vi "KillCamera.vi"(11 "Camera":T1) -> ()   [LabVIEW 2015]
uses:
  ROS/Code/SubVIs/BaxterCamera.ctl
  ROS/Code/_ROSDefinition.vi
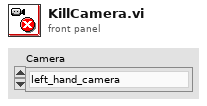
[diagram p1: front panel]
types:
  T1 = typedef "BaxterCamera.ctl" = enum16{"left_hand_camera", "right_hand_camera", "head_camera"}
  T2 = typedef "_ROSControl.ctl" = cluster{"topic port":u16, "Node":string, "topic":string, "type":string, "node port":u16, "error ":errorcluster, "Direction":T3, "Update (ms)":u16, "FIFO size":u16}
  T3 = typedef "_ROSDirection.ctl" = enum16{"Node", "Publisher", "Subscriber", "ServiceClient", "ServiceProvider"}
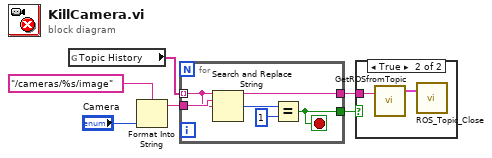
[diagram p0: block diagram]
diagram:
  n1 = global read "_ROSDefinition.vi" "Topic History"() -> (w3:string[])
  n2 = Format Into String(format string="/cameras/%s/image" ("topic"), "Camera") -> (resulting string=w4:string)  [unwired: 2 in, 1 out]
  n3 = for {
    tunnel: w3 -> [w11] mode=indexing
    tunnel: w4 -> [w12]
    tunnel: [w8] -> w5
    tunnel: [w7] -> w6
    stop <- w7 stop-if-true
    n4 = Search and Replace String(input string=w11, search string=w12, replace string=w11) -> (result string=w8:string, number of replacements=w10:i32)  [unwired: 5 in, 2 out]
    n5 = Equal?(x=w10, y=1) -> (x = y?=w7:bool)
  }
  n6 = case shown="True" w6 {
    tunnel: w5 -> [_ w13]
    frame False {
    }
    frame True {
      n7 = call "GetROSfromTopic.vi"("Topic"=w13) -> ("ROS"=w14:T2)  [unwired: 1 in, 2 out]
      n8 = call "ROS_Topic_Close.vi"("ROS in"=w14) -> ()  [unwired: 3 in, 1 out]
    }
  }
